vi "Test Client.vi"() -> ()   [LabVIEW 2020]
uses:
  c835d68e-6a3e-4298-b2e5-62dd2310970f.vi
  ee8d1fbd-e618-4e25-9b4e-a02f87d51e48.vi
  source/Client/Client/Client.lvclass
panel:
  in  "Put value":i64
  in  "update (ms)":i32=100
  in  "stop":bool
  out "Map":map{string, variant}(c390)
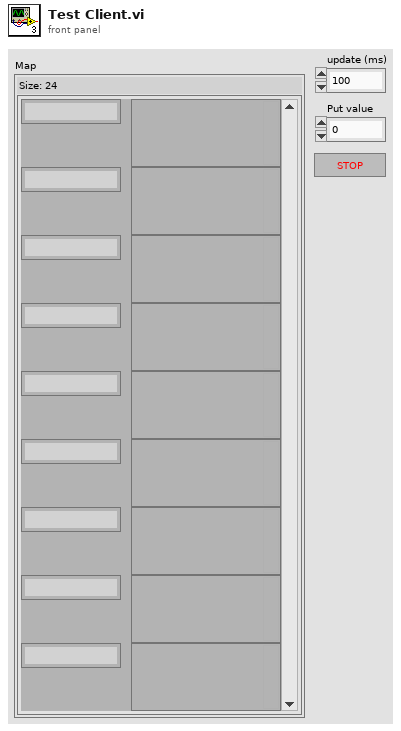
[diagram p1: front panel]
types:
  T1 = typedef "Value.lvlib/Type Code.ctl" = enum8{"Null", "Bool", "BoolA", "Int8", "Int8A", "Int16", "Int16A", "Int32", "Int32A", "Int64", "Int64A", "UInt8", "UInt8A", "UInt16", "UInt16A", "UInt32", "UInt32A", "UInt64", "UInt64A", "Float32", "Float32A", "Float64", "Float64A", "String", "StringA", "Struct", "StructA", "Union", "UnionA", "Any", "AnyA"}
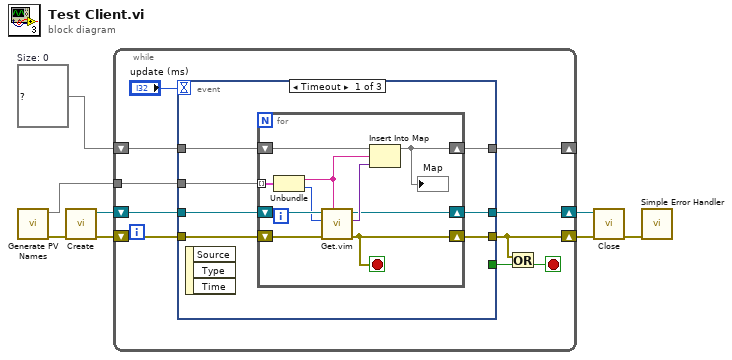
[diagram p0: block diagram]
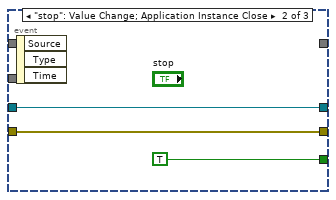
[diagram p2: hidden frame]
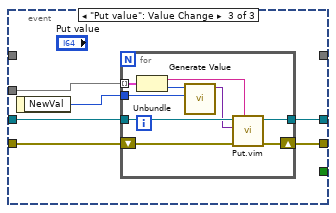
[diagram p3: hidden frame]
diagram:
  w4 = map{string, variant} {}  # Size: 0
  n1 = call "Generate PV Names.vi"() -> ("error out"=w3:errorcluster, "map"=w2:map{string, T1})  [unwired: 10 in]
  n2 = call "Create.vi"("error in (no error)"=w3) -> ("error out"=w8:errorcluster, "Client out"=w7:refnum<class "Client.lvclass">)  [unwired: 9 in]
  n3 = while {
    tunnel: w2 -> [w17]
    shift-right: [w12] -> w6
    shift-left: w8 -> [w13]
    shift-right: [w11] -> w5
    shift-left: w7 -> [w14]
    shift-right: [w16] -> _
    shift-left: w4 -> [w18]
    stop <- w15 stop-if-true
    n4 = event shown="[0] Timeout" {
      selector: _ -> [_ _ _]
      dyn-events: _ -> [_ _ _]
      timeout: "update (ms)" -> [_ _ _]
      tunnel: w18 -> [w25 _ _]
      tunnel: w17 -> [w24 _ w44]
      tunnel: [w23 _ _] -> w16
      tunnel: w14 -> [w22 w36 w42]
      tunnel: w13 -> [w21 w37 w41]
      tunnel: [w20 w37 w40] -> w12
      tunnel: [w19 w36 w39] -> w11
      tunnel: [_ TRUE ("stop") _] -> w10
      event Timeout {
        n5 = event-data() -> ()  [unwired: 1 in, 3 out]
        n6 = for {
          shift-right: [w35] -> w23
          shift-left: w25 -> [w29]
          tunnel: w24 -> [w34] mode=indexing
          shift-right: [w27] -> w20
          shift-left: w21 -> [w33]
          shift-right: [w28] -> w19
          shift-left: w22 -> [w32]
          stop <- w27 stop-if-true
          n7 = Unbundle(w34) -> (w30:string, "Enum"=w26:T1)
          n8 = call "Get.vim"("PV name"=w30, "error in"=w33, "default"=w26, "Client in"=w32) -> ("error out"=w27:errorcluster, "value"=w31:variant, "Client out"=w28:refnum<class "Client.lvclass">)  [unwired: 3 in, 2 out]
          n9 = Insert Into Map(map in=w29, key=w30, value=w31) -> (map out=w35:map{string, variant})  [unwired: 2 out]
          "Map" <- w35
        }
      }
      event "stop": Value Change; Application Instance Close {
        n10 = event-data() -> ()  [unwired: 1 in, 3 out]
      }
      event "Put value": Value Change {
        n11 = event-data() -> ("NewVal"=w43:i64)  [unwired: 1 in]
        n12 = for {
          tunnel: w42 -> [w50]
          tunnel: [w51] -> w39
          shift-right: [w52] -> w40
          shift-left: w41 -> [w53]
          tunnel: w44 -> [w49] mode=indexing
          tunnel: w43 -> [w47]
          n13 = Unbundle(w49) -> (w46:string, "Enum"=w48:T1)
          n14 = call "Generate Value.vi"("base value"=w47, "type code"=w48) -> ("value"=w45:variant)  [unwired: 9 in]
          n15 = call "Put.vim"("PV name"=w46, "error in"=w53, "value in"=w45, "Client in"=w50) -> ("error out"=w52:errorcluster, "Client out"=w51:refnum<class "Client.lvclass">)  [unwired: 4 in, 2 out]
        }
      }
    }
    n16 = Or(x=w12, y=w10) -> (x .or. y?=w15:bool)
  }
  n17 = call "Close.vi"("error in (no error)"=w6, "Client in"=w5) -> ("error out"=w1:errorcluster)  [unwired: 9 in]
  n18 = call <vilib>:"Simple Error Handler.vi"("error in (no error)"=w1) -> ()  [unwired: 4 in, 5 out]
